vi "all.vi"() -> ()   [LabVIEW 2025]
uses:
  <vilib>/Utility/error.llb/Trim Whitespace One-Sided.vi
  Sort 2D Array (numeric).vi
panel:
  in  "Open panels":bool
  in  "Open diagrams":bool
  out "VIs":string
  in  "?":bool
  # "This VI is a tool for saving all model support or project VIs to a previous version.\nIt is not used by the standard process model; It doesn't matter if it is broken.\nYou can ignore it or delete it from your project if you like."
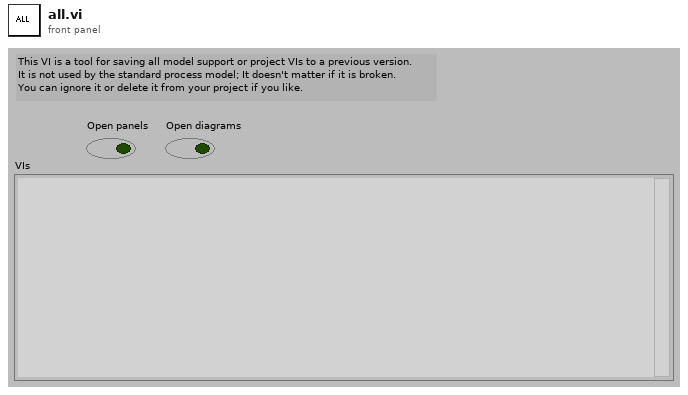
[diagram p1: front panel]
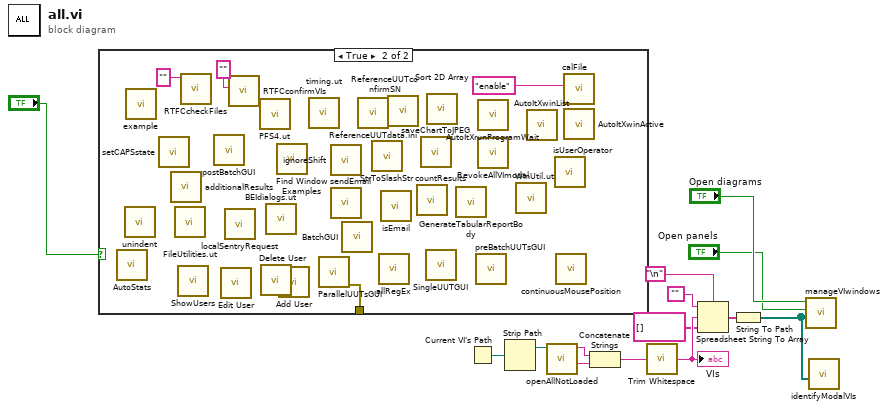
[diagram p0: block diagram]
diagram:
  n1 = case shown="True" "?" {
    tunnel: [_ w18] -> _
    frame False {
    }
    frame True {
      n2 = call "AutoStats.vi"() -> ()  [unwired: 2 in, 10 out]
      n3 = call "unindent.vi"() -> ()  [unwired: 1 in, 11 out]
      n4 = call "example.vi"() -> ()  [unwired: 1 in]
      n5 = call "setCAPSstate.vi"() -> ()  [unwired: 11 in, 1 out]
      n6 = call "additionalResults.vi"() -> ()  [unwired: 9 in, 3 out]
      n7 = call "FileUtilities.ut.vi"() -> ()  [unwired: 12 out]
      n8 = call "ShowUsers.vi"() -> ()  [unwired: 4 in, 1 out]
      n9 = call "RTFCcheckFiles.vi"("SW file Spec string"="") -> ()  [unwired: 8 in, 3 out]
      n10 = call "postBatchGUI.vi"() -> ()  [unwired: 10 in, 2 out]
      n11 = call "Edit User.vi"() -> ()  [unwired: 4 in, 1 out]
      n12 = call "localSentryRequest.vi"() -> ()  [unwired: 4 in, 8 out]
      n13 = call "RTFCconfirmVIs.vi"("VIpaths"="") -> ()  [unwired: 8 in, 3 out]
      n14 = call "PFS4.ut.vi"() -> ()  [unwired: 12 out]
      n15 = call "Delete User.vi"() -> ()  [unwired: 4 in, 1 out]
      n16 = call "BEIdialogs.ut.vi"() -> ()  [unwired: 12 out]
      n17 = call "Find Window Examples.vi"() -> ()  [unwired: 1 in]
      n18 = call "Add User.vi"() -> ()  [unwired: 4 in, 1 out]
      n19 = call "timing.ut.vi"() -> ()  [unwired: 12 out]
      n20 = call "ParallelUUTsGUI.vi"() -> ("error out"=w18:errorcluster)  [unwired: 1 in, 10 out]
      n21 = call "ignoreShift.vi"() -> ()  [unwired: 1 in]
      n22 = call "sendEmail.vi"() -> ()  [unwired: 11 in, 1 out]
      n23 = call "BatchGUI.vi"() -> ()  [unwired: 11 in, 1 out]
      n24 = call "ReferenceUUTdata.ini.vi"() -> ()  [unwired: 10 in, 2 out]
      n25 = call "StrToSlashStr.vi"() -> ()  [unwired: 10 in, 2 out]
      n26 = call "allRegEx.vi"() -> ()  [unwired: 1 out]
      n27 = call "isEmail.vi"() -> ()  [unwired: 1 in, 11 out]
      n28 = call "ReferenceUUTconfirmSN.vi"() -> ()  [unwired: 10 in, 2 out]
      n29 = call "countResults.vi"() -> ()  [unwired: 11 in, 1 out]
      n30 = call "saveChartToJPEG.vi"() -> ()  [unwired: 11 in, 1 out]
      n31 = call "SingleUUTGUI.vi"() -> ()  [unwired: 1 in, 11 out]
      n32 = call-poly "Sort 2D Array.vi"() -> ()  [unwired: 5 in, 2 out]
      n33 = call "GenerateTabularReportBody.vi"() -> ()  [unwired: 10 in, 2 out]
      n34 = call "preBatchUUTsGUI.vi"() -> ()  [unwired: 7 in, 5 out]
      n35 = call "AutoItXrunProgramWait.vi"() -> ()  [unwired: 11 in, 1 out]
      n36 = call "RevokeAllVImodal.vi"() -> ()  [unwired: 11 in, 1 out]
      n37 = call "WinUtil.ut.vi"() -> ()  [unwired: 2 in]
      n38 = call "AutoItXwinList.vi"() -> ()  [unwired: 10 in, 2 out]
      n39 = call "isUserOperator.vi"() -> ()  [unwired: 11 in, 1 out]
      n40 = call "continuousMousePosition.vi"() -> ()  [unwired: 1 in]
      n41 = call "calFile.vi"("key"="enable") -> ()  [unwired: 7 in, 4 out]
      n42 = call "AutoItXwinActive.vi"() -> ()  [unwired: 9 in, 3 out]
    }
  }
  n43 = Current VI's Path() -> (path=w13:path)
  n44 = Strip Path(path=w13) -> (stripped path=w12:path)  [unwired: 1 out]
  n45 = call "openAllNotLoaded.vi"("path"=w12) -> ("UnLoaded VIs opened"=w10:string, "VIs at path heirarchy"=w11:string)  [unwired: 7 in, 2 out]
  n46 = Concatenate Strings(w11, w10) -> (w9:string)
  n47 = call <vilib>:"Trim Whitespace.vi"("string"=w9) -> ("trimmed string"=w5:string)  [unwired: 1 in]
  "VIs" <- w5
  n48 = Spreadsheet String To Array(delimiter (Tab)="\n", format string="", spreadsheet string=w5, array type (2D Dbl)=string[] []) -> (array=w6:string[])
  n49 = String To Path(string=w6) -> (path=w1:path[])
  n50 = call "manageVIwindows.vi"("Files"=w1, "Open panels"="Open panels", "Open diagrams"="Open diagrams") -> ()  [unwired: 8 in, 1 out]
  n51 = call "identifyModalVIs.vi"("Files"=w1) -> ()  [unwired: 10 in, 1 out]
